vi "Apply.vi"(8 "Error In":errorcluster, 11 "object in":refnum<class "Continuous Waveform Acq CFG.lvclass">) -> (0 "Error Out":errorcluster, 3 "object out":refnum<class "Continuous Waveform Acq CFG.lvclass">)   [LabVIEW 2023, in "PXIe-5172 Simulated.lvlib" / "Continuous Waveform Acq CFG.lvclass"]
uses:
  Continuous Waveform Acq CFG.lvclass
  Continuous Waveform Acq CFG.lvclass/Continuous Waveform Acq CFG.ctl
  <instrlib>/niScope/Utility/niScope Get Channel Name From String.vi
  <instrlib>/niScope/Configure/Trigger/niScope Configure Trigger Immediate.vi
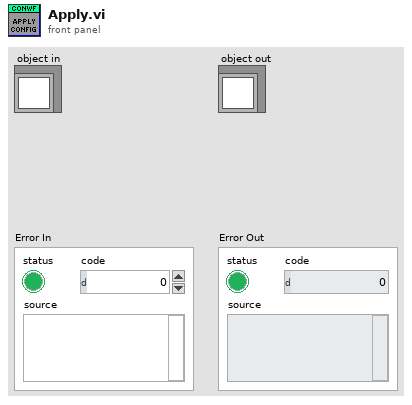
[diagram p1: front panel]
types:
  T1 = cluster{"HW Device Name":string, "Resouce Identifier":string, "Options String":string, "Channels":string, "Vertical Range":dbl, "Vertical Offset":dbl, "Vertical Coupling":i32, "Input Impedance":u32, "Min Sample Rate":dbl}
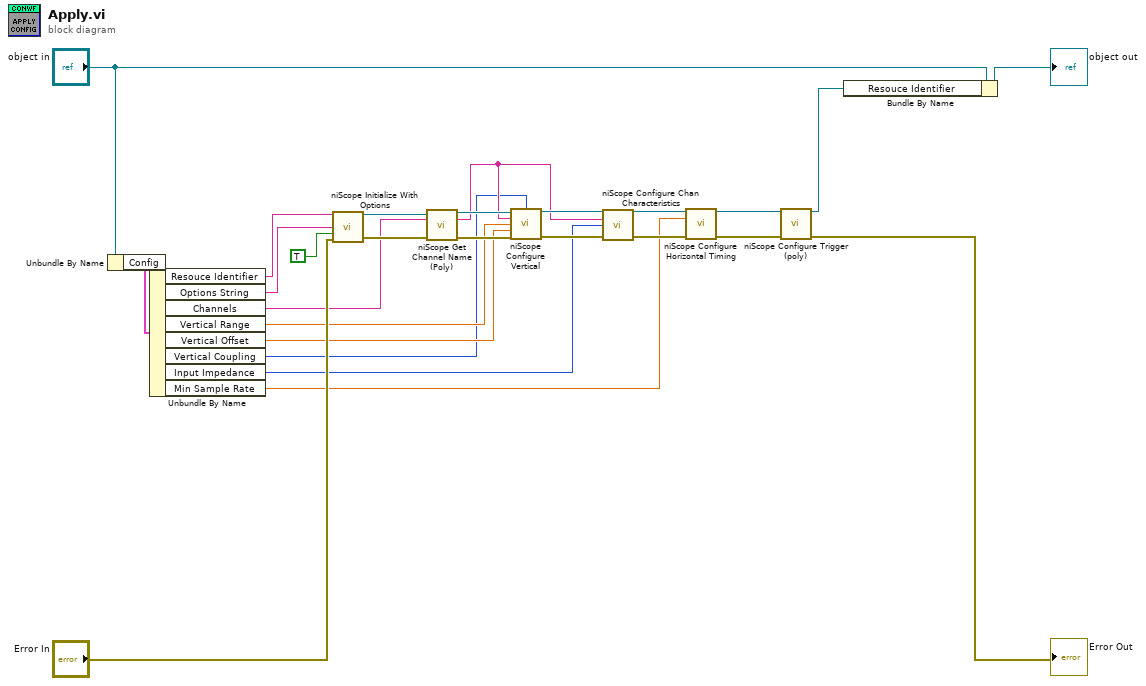
[diagram p0: block diagram]
diagram:
  n1 = Unbundle By Name("object in") -> ("Config"=w3:T1)
  n2 = Unbundle By Name(w3) -> ("Resouce Identifier"=w2:string, "Options String"=w1:string, "Channels"=w11:string, "Vertical Range"=w10:dbl, "Vertical Offset"=w9:dbl, "Vertical Coupling"=w8:i32, "Input Impedance"=w7:u32, "Min Sample Rate"=w6:dbl)
  n3 = call <instrlib>:"niScope Initialize With Options.vi"("resource name"=w2, "option string"=w1, "reset device"=TRUE, "error in"="Error In") -> ("instrument handle"=w19:refnum<k15>, "error out"=w20:errorcluster)  [unwired: 10 in]
  n4 = call-poly <instrlib>:"niScope Get Channel Name (Poly).vi"("instrument handle"=w19, "index"=w11, "error in"=w20) -> ("instrument handle out"=w18:refnum<k15>, "channel name"=w12:string, "error out"=w17:errorcluster)  [unwired: 10 in]
  n5 = call <instrlib>:"niScope Configure Vertical.vi"("instrument handle"=w18, "vertical coupling"=w8, "channels"=w12, "vertical range"=w10, "vertical offset"=w9, "error in"=w17) -> ("instrument handle out"=w16:refnum<k15>, "error out"=w15:errorcluster)  [unwired: 8 in]
  n6 = call <instrlib>:"niScope Configure Chan Characteristics.vi"("instrument handle"=w16, "channels"=w12, "input impedance"=w7, "error in"=w15) -> ("instrument handle out"=w14:refnum<k15>, "error out"=w13:errorcluster)  [unwired: 10 in]
  n7 = call <instrlib>:"niScope Configure Horizontal Timing.vi"("instrument handle"=w14, "min sample rate"=w6, "error in"=w13) -> ("instrument handle out"=w4:refnum<k15>, "error out"=w5:errorcluster)  [unwired: 11 in]
  n8 = call-poly <instrlib>:"niScope Configure Trigger (poly).vi"("instrument handle"=w4, "error in"=w5) -> ("instrument handle out"=w22:refnum<k15>, "error out"=→"Error Out":errorcluster)  [unwired: 12 in]
  n9 = Bundle By Name(cluster="object in", "Resouce Identifier"=w22) -> (→"object out":refnum<class "Continuous Waveform Acq CFG.lvclass">)
